vi "DHE_Setbpp.vi"(2 "DHE_bpp":i32) -> ()   [LabVIEW 2016]
uses:
  private/vis/DHE_GBLDriverVariables.vi
  DBSHAND/private/vis/DatabaseHand_Element_Set(I32).vi
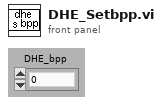
[diagram p1: front panel]
types:
  T1 = typedef "DatabaseHand_RefNum.ctl" = refnum<vi>
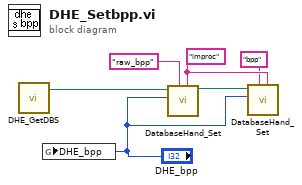
[diagram p0: block diagram]
diagram:
  w3 = "improc" ("group")
  n1 = call "DHE_GetDBS.vi"() -> ("DHE_DBSRef"=w6:T1)  [unwired: 9 out]
  n2 = global write "DHE_GBLDriverVariables.vi" "DHE_bpp"("DHE_bpp") -> ()
  n3 = call-poly "DatabaseHand_Set.vi"("group"=w3, "name"="raw_bpp", "value"="DHE_bpp", "Database RefNum in"=w6) -> ("Database RefNum out"=w4:T1)  [unwired: 4 in, 3 out]
  n4 = call-poly "DatabaseHand_Set.vi"("group"=w3, "name"="bpp", "value"="DHE_bpp", "Database RefNum in"=w4) -> ()  [unwired: 4 in, 4 out]
